vi "Calculate Hysteresis.vi"(8 "error in (no error)":errorcluster, 9 "SensorID":i32, 10 "FS Sensors":T1[](array[typedef]), 11 "Calibration Points":T3[](array[typedef])) -> (0 "error out":errorcluster, 2 "Max Hysteresis":dbl, 3 "Hysteresis Results":T2[](array[typedef]))   [LabVIEW 2026, in "Analysis.lvlib"]
uses:
  Analysis.lvlib
  controls/Messaging Payloads/Calibration Point Table Insert.ctl
  Hysteresis Result.ctl
  Full Scale Sensor Cluster.ctl
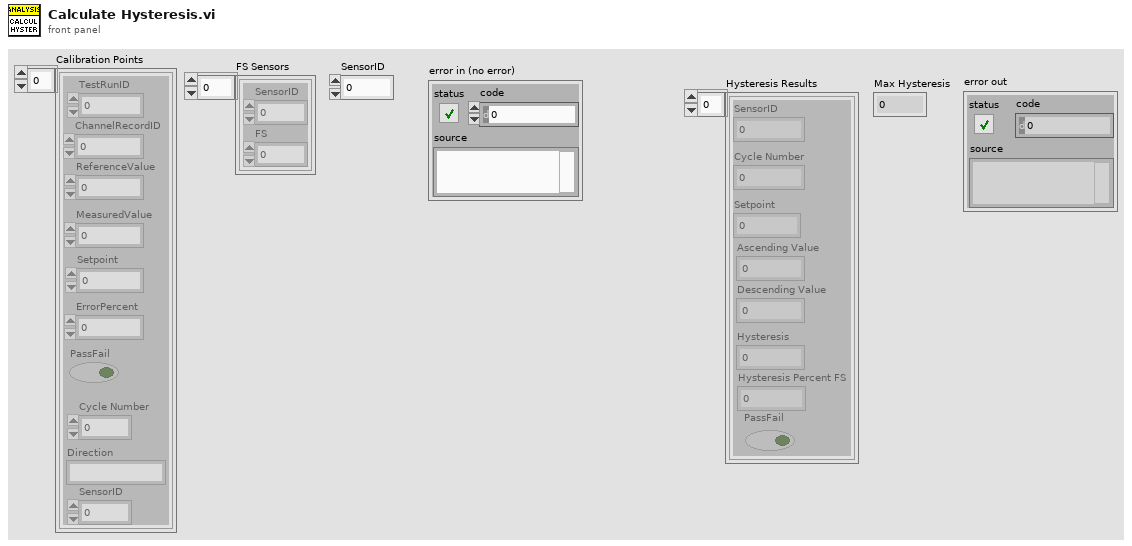
[diagram p1: front panel]
types:
  T1 = typedef "Analysis.lvlib/Full Scale Sensor Cluster.ctl" = cluster{"SensorID":i32, "FS":dbl}
  T2 = typedef "Analysis.lvlib/Hysteresis Result.ctl" = cluster{"Setpoint":dbl, "Ascending Value":dbl, "Cycle Number":i32, "SensorID":i32, "Descending Value":dbl, "Hysteresis":dbl, "Hysteresis Percent FS":dbl, "PassFail":bool}
  T3 = typedef "Calibration Point Table Insert.ctl" = cluster{"TestRunID":i32, "ChannelRecordID":i32, "Setpoint":dbl, "MeasuredValue":dbl, "ErrorPercent":dbl, "PassFail":bool, "ReferenceValue":dbl, "Cycle Number":i32, "Direction":string, "SensorID":i32}
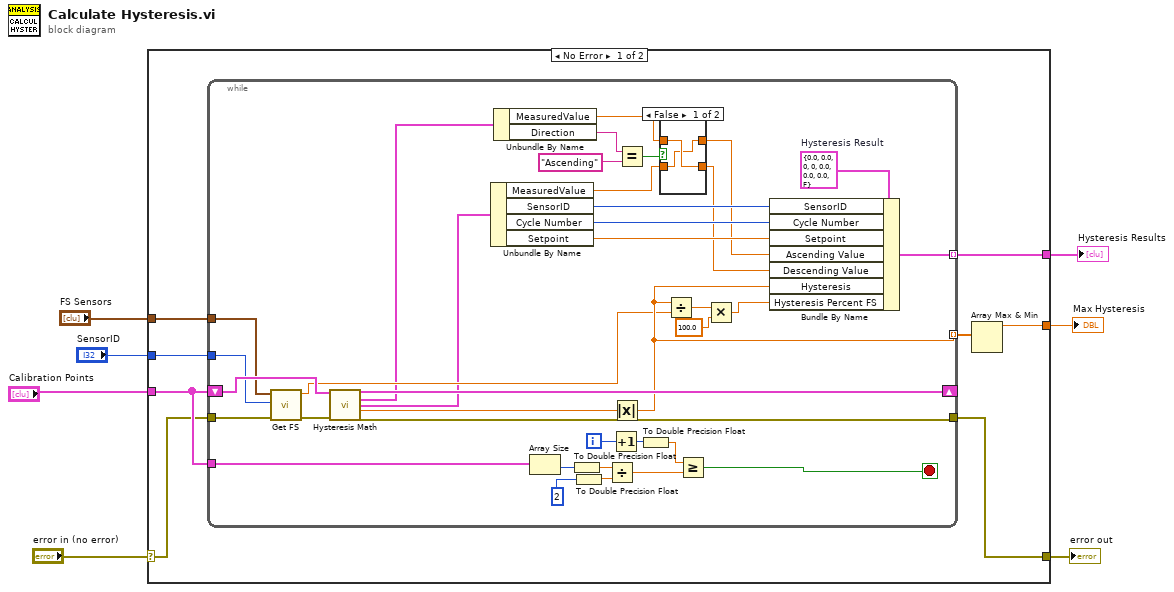
[diagram p0: block diagram]
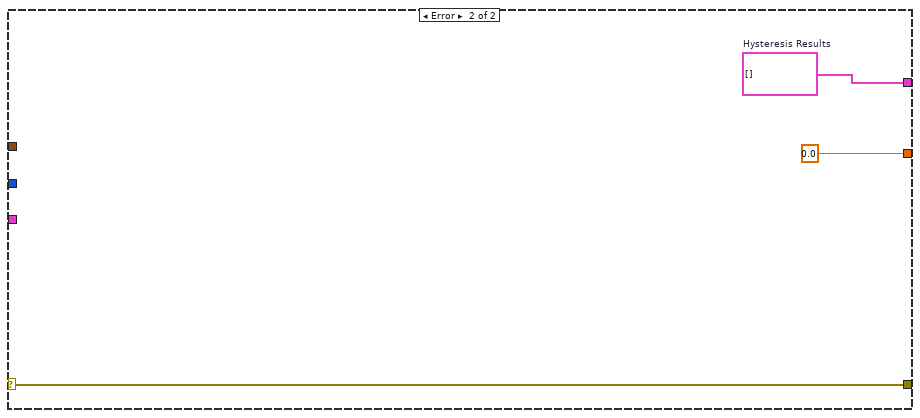
[diagram p3: hidden frame]
diagram:
  n1 = case shown="No Error" "error in (no error)" {
    selector: "error in (no error)" -> [w11 w59]
    tunnel: "Calibration Points" -> [w15 _]
    tunnel: [w10 w59] -> w6
    tunnel: [w12 w58] -> w4
    tunnel: [w13 0.0] -> w3
    tunnel: "FS Sensors" -> [w9 _]
    tunnel: "SensorID" -> [w8 _]
    frame No Error {
      n2 = while {
        shift-right: [w29] -> _
        shift-left: w15 -> [w28]
        tunnel: w15 -> [w45]
        tunnel: [w41] -> w12 mode=indexing
        tunnel: [w19] -> w14 mode=indexing
        tunnel: w11 -> [w27]
        tunnel: [w25] -> w10
        tunnel: w9 -> [w24]
        tunnel: w8 -> [w23]
        i -> [w44]
        stop <- w46 stop-if-true
        w42 = T2 {"Setpoint"=0.0, "Ascending Value"=0.0, "Cycle Number"=0, "SensorID"=0, "Descending Value"=0.0, "Hysteresis"=0.0, "Hysteresis Percent FS"=0.0, "PassFail"=FALSE}  # Hysteresis Result
        n3 = call "Get FS.vi"("error in (no error)"=w27, "SensorID"=w23, "FS Sensors"=w24) -> ("error out"=w26:errorcluster, "FS"=w18:dbl)  [unwired: 7 in]
        n4 = call "Hysteresis Math.vi"("Calibration Points in"=w28, "error in (no error)"=w26) -> ("Calibration Points out"=w29:T3[], "Current Calibration Point"=w17:T3, "Next Calibration Point"=w16:T3, "Hysteresis"=w30:dbl, "error out"=w25:errorcluster)  [unwired: 9 in]
        n5 = Unbundle By Name(w16) -> ("MeasuredValue"=w33:dbl, "SensorID"=w40:i32, "Cycle Number"=w39:i32, "Setpoint"=w38:dbl)
        n6 = Unbundle By Name(w17) -> ("MeasuredValue"=w34:dbl, "Direction"=w37:string)
        n7 = Array Size(array=w45) -> (size(s)=w50:i32)
        n8 = To Double Precision Float(number=w50) -> (double precision float=w49:dbl)
        n9 = To Double Precision Float(number=2 ("index")) -> (double precision float=w47:dbl)
        n10 = Divide(x=w49, y=w47) -> (x/y=w52:dbl)
        n11 = Increment(x=w44) -> (x+1=w43:i32)
        n12 = Absolute Value(x=w30) -> (abs(x)=w19:dbl)
        n13 = Equal?(x=w37, y="Ascending" ("x")) -> (x = y?=w35:bool)
        n14 = To Double Precision Float(number=w43) -> (double precision float=w51:dbl)
        n15 = case shown="False" w35 {
          tunnel: w34 -> [w54 w56]
          tunnel: [w53 w56] -> w32
          tunnel: w33 -> [w53 w55]
          tunnel: [w54 w55] -> w31
          frame False {
          }
          frame True {
          }
        }
        n16 = Divide(x=w19, y=w18) -> (x/y=w22:dbl)
        n17 = Greater Or Equal?(x=w51, y=w52) -> (x >= y?=w46:bool)
        n18 = Multiply(x=w22, y=100.0) -> (x*y=w20:dbl)
        n19 = Bundle By Name(cluster=w42, "SensorID"=w40, "Cycle Number"=w39, "Setpoint"=w38, "Ascending Value"=w32, "Descending Value"=w31, "Hysteresis"=w19, "Hysteresis Percent FS"=w20) -> (w41:T2)
      }
      n20 = Array Max & Min(array=w14) -> (max value=w13:dbl)  [unwired: 3 out]
    }
    frame Error {
      w58 = T2[] []  # Hysteresis Results
    }
  }
  "error out" <- w6
  "Hysteresis Results" <- w4
  "Max Hysteresis" <- w3
